vi "Write FP Control.vi"(8 "error in (no error)":errorcluster, 9 "Control Value":variant, 10 "Control Name":string="Configuration", 11 "Measure Object in":refnum<class "Measure Object.lvclass">) -> (0 "error out":errorcluster, 3 "Measure Object out":refnum<class "Measure Object.lvclass">)   [LabVIEW 2015, in "Measure Object.lvclass"]
uses:
  Measure Object.lvclass
  Measure Object.lvclass/Measure Object.ctl
  Read Front Panel ref.vi
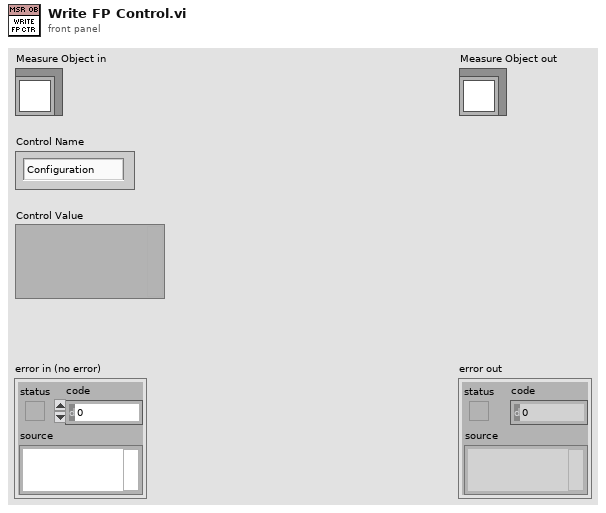
[diagram p1: front panel]
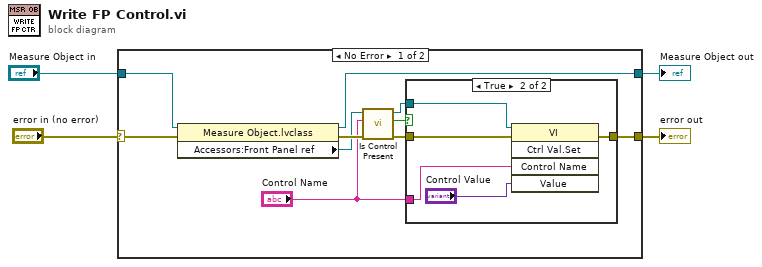
[diagram p0: block diagram]
diagram:
  n1 = case shown="No Error" "error in (no error)" {
    selector: "error in (no error)" -> [w14 w22]
    tunnel: [w11 w22] -> w3
    tunnel: [w12 w21] -> w1
    tunnel: "Measure Object in" -> [w13 w21]
    frame No Error {
      n2 = property class="Measure Object.lvclass"(reference=w13, error in=w14) -> (reference out=w12:refnum<class "Measure Object.lvclass">, error out=w10:errorcluster, "Accessors:Front Panel ref"=w8:refnum<vi>)
      n3 = call "Is Control Present.vi"("Error In"=w10, "Control label"="Control Name", "VI ref"=w8) -> ("Error Out"=w9:errorcluster, "Present"=w5:bool, "VI ref out"=w7:refnum<vi>)  [unwired: 6 in]
      n4 = case shown="True" w5 {
        tunnel: [w15 w20] -> w11
        tunnel: w9 -> [w15 w19]
        tunnel: w7 -> [_ w18]
        tunnel: "Control Name" -> [_ w17]
        frame False {
        }
        frame True {
          n5 = invoke class="VI" method="Ctrl Val.Set"(reference=w18, error in=w19, "Control Name"=w17, "Value"="Control Value") -> (error out=w20:errorcluster)  [unwired: 1 in, 4 out]
        }
      }
    }
    frame Error {
    }
  }
  "error out" <- w3
  "Measure Object out" <- w1
